vi "Bits To Bytes.vi"(1 "Bits":bool[](array[boolean])) -> (0 "Bytes":u8[](array[numeric]))   [LabVIEW 2020]
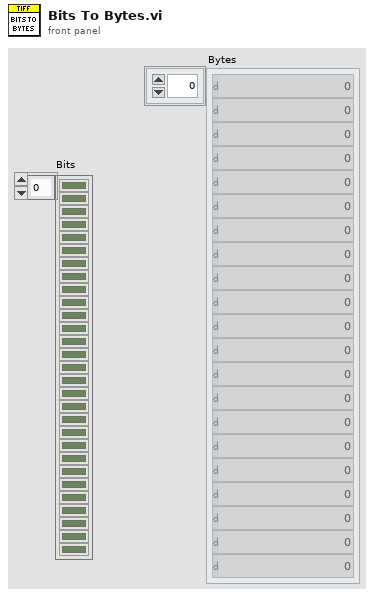
[diagram p1: front panel]
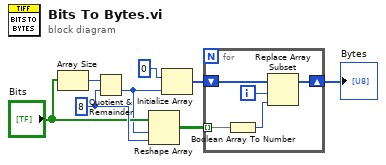
[diagram p0: block diagram]
diagram:
  w6 = 8 ("y")
  n1 = Array Size(array="Bits") -> (size(s)=w8:i32)
  n2 = Quotient & Remainder(x=w8, y=w6) -> (floor(x/y)=w1:i32)  [unwired: 1 out]
  n3 = Reshape Array("Bits", w1, w6) -> (w2:bool[][])
  n4 = Initialize Array(u8 0, w1) -> (w5:u8[])
  n5 = for {
    tunnel: w2 -> [w13] mode=indexing
    shift-right: [w11] -> w4
    shift-left: w5 -> [w12]
    i -> [w10]
    n6 = Boolean Array To Number(Boolean array=w13) -> (number=w9:u8)
    n7 = Replace Array Subset(array=w12, new element=w9, index=w10) -> (w11:u8[])
  }
  "Bytes" <- w4
